vi "potential-field.vi"(10 "Debug":bool=TRUE, 11 "IA State Output in":T1={"our_robots"=[], "enemy_robots"=[], "balls"=[], "geometry"={"line_width"=0, "field_length"=0, "field_width"=0, "boundary_width"=0, "referee_width"=0, "goal_width"=0, "goal_depth"=0, "goal_wall_width"=0, "center_circle_radius"=0, "defense_radius"=0, "defense_stretch"=0, "free_kick_from_defense_dist"=0, "penalty_spot_from_field_line_dist"=0, "penalty_line_from_spot_dist"=0}, "IA Judge"={"stage"="", "command"="", "our_goalie_id"=0.0, "enemy_goalie_id"=0.0, "command enum"=enum."Halt", "Time"=enum."Azul"}, "Received Timestamp"=timestamp(0 s since 1904-01-01), "Events"={"Touch"=FALSE, "Ball out"=FALSE, "id touch"=0.0, "Ball out of \nVision"=FALSE, "Ball inside \nGoalie area"=FALSE, "Robot not responding"=FALSE, "Robots responding status"=[1.0, 1.0, 1.0, 1.0, 1.0, 1.0], "Enemy Ball \nPossession"=FALSE, "Pass State"=FALSE, "id end of pass"=0.0, "Kick"=FALSE, "Id ini Possession"=0.0, "Ball Possesion"=FALSE, "Id Possesion"=0.0}}) -> (3 "IA State Output out":T1={"our_robots"=[], "enemy_robots"=[], "balls"=[], "geometry"={"line_width"=0, "field_length"=0, "field_width"=0, "boundary_width"=0, "referee_width"=0, "goal_width"=0, "goal_depth"=0, "goal_wall_width"=0, "center_circle_radius"=0, "defense_radius"=0, "defense_stretch"=0, "free_kick_from_defense_dist"=0, "penalty_spot_from_field_line_dist"=0, "penalty_line_from_spot_dist"=0}, "IA Judge"={"stage"="", "command"="", "our_goalie_id"=0.0, "enemy_goalie_id"=0.0, "command enum"=enum."Halt", "Time"=enum."Azul"}, "Received Timestamp"=timestamp(0 s since 1904-01-01), "Events"={"Touch"=FALSE, "Ball out"=FALSE, "id touch"=0.0, "Ball out of \nVision"=FALSE, "Ball inside \nGoalie area"=FALSE, "Robot not responding"=FALSE, "Robots responding status"=[1.0, 1.0, 1.0, 1.0, 1.0, 1.0], "Enemy Ball \nPossession"=FALSE, "Pass State"=FALSE, "id end of pass"=0.0, "Kick"=FALSE, "Id ini Possession"=0.0, "Ball Possesion"=FALSE, "Id Possesion"=0.0}})   [LabVIEW 2018]
uses:
  Core/AI Input.ctl
  Core/AI Robot.ctl
  Intel/Functions Enum.ctl
  Intel/AttackerStates.ctl
  Core/AI Ball.ctl
  Core/Field Size.ctl
  Core/AI Judge.ctl
  Intel/Command Enum.ctl
  Util/Events/Events.ctl
  <vilib>/Analysis/_algsub.llb/Vector Norm Type.ctl
  <vilib>/Analysis/_algsub.llb/Real Vector Norm.vi
  <vilib>/Analysis/coordinate.llb/2D Cartesian Coordinate Rotation (Scalar).vi
  <vilib>/Analysis/NI_AALPro.lvlib
panel:
  in  "influence radius":dbl=500.0 format="%#_13g"
  in  "multiplier":dbl(slide)=1.0 scale=0.0..10.0
  in  "dist to nullify pot field":dbl=800.0 format="%#_13g"
  in  "min dist to reduce":dbl=500.0 format="%#_13g"
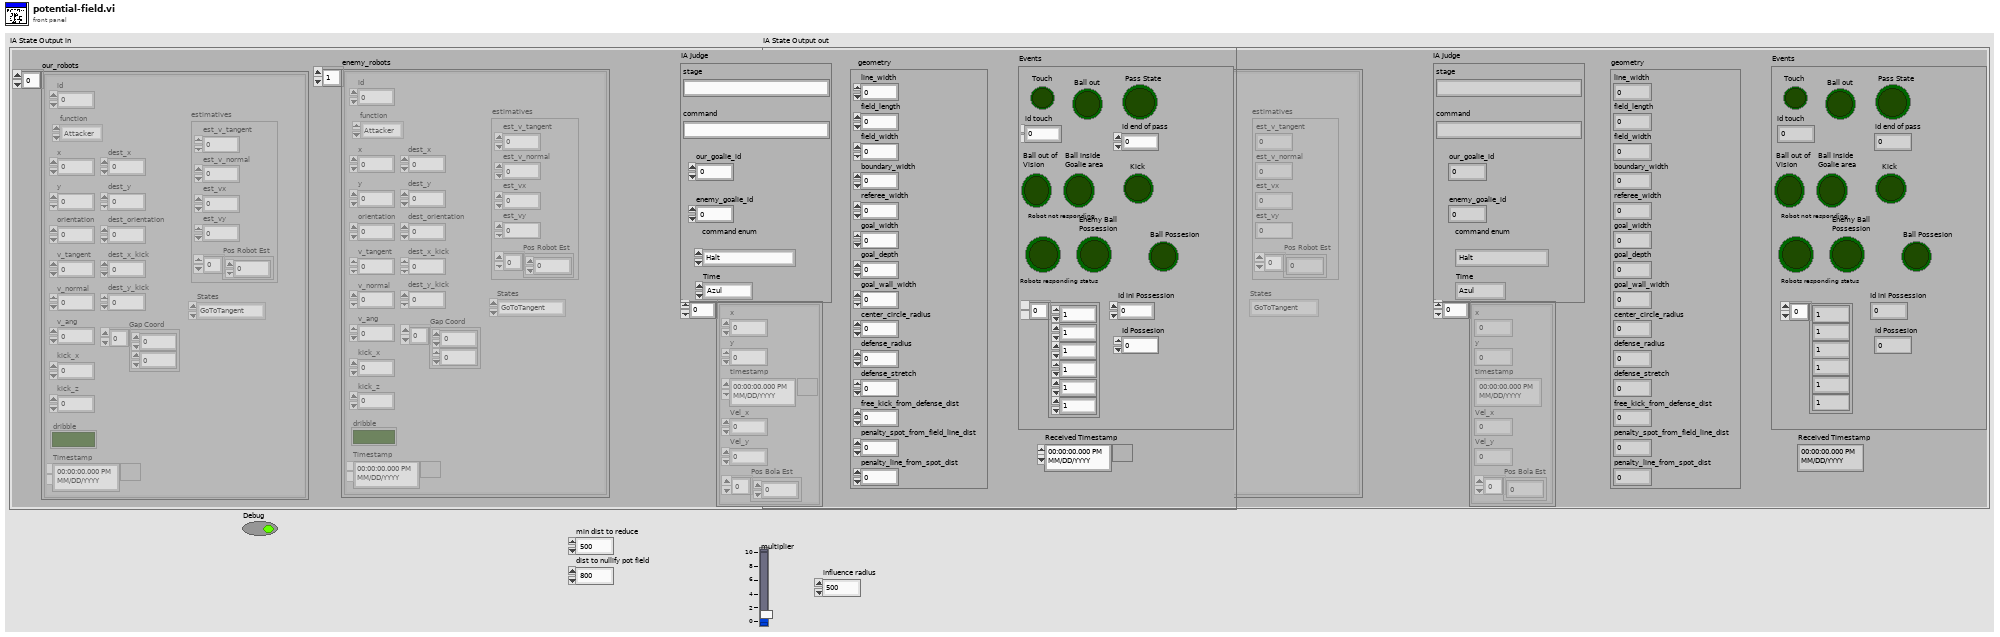
[diagram p1: front panel]
types:
  T1 = typedef "AI Input.ctl" = cluster{"our_robots":T2[], "enemy_robots":T2[], "balls":T5[], "geometry":T6, "IA Judge":T7, "Received Timestamp":timestamp, "Events":T9}
  T2 = typedef "AI Robot.ctl" = cluster{"id":u32, "function":T3, "x":dbl, "y":dbl, "orientation":dbl, "v_tangent":dbl, "v_normal":dbl, "v_ang":dbl, "kick_x":dbl, "kick_z":dbl, "dribble":bool, "Timestamp":timestamp, "dest_x":dbl, "dest_y":dbl, "dest_orientation":dbl, "estimatives":cluster{"est_v_tangent":dbl, "est_v_normal":dbl, "est_vx":dbl, "est_vy":dbl, "Pos Robot Est":dbl[]}, "dest_x_kick":dbl, "dest_y_kick":dbl, "Gap Coord":dbl[], "States":T4}
  T3 = typedef "Functions Enum.ctl" = enum16{"Attacker", "Goalie", "Defender", "Striker", "Goto 0", "Dummy", "Kicker", "ZigZag"}
  T4 = typedef "AttackerStates.ctl" = enum16{"Pass", "GoToTangent", "BallGetting", "GoToKick", ""}
  T5 = typedef "AI Ball.ctl" = cluster{"x":dbl, "y":dbl, "timestamp":timestamp, "Vel_x":dbl, "Vel_y":dbl, "Pos Bola Est":dbl[]}
  T6 = typedef "Field Size.ctl" = cluster{"line_width":u32, "field_length":u32, "field_width":u32, "boundary_width":u32, "referee_width":u32, "goal_width":u32, "goal_depth":u32, "goal_wall_width":u32, "center_circle_radius":u32, "defense_radius":u32, "defense_stretch":u32, "free_kick_from_defense_dist":u32, "penalty_spot_from_field_line_dist":u32, "penalty_line_from_spot_dist":u32}
  T7 = typedef "AI Judge.ctl" = cluster{"stage":string, "command":string, "our_goalie_id":dbl, "enemy_goalie_id":dbl, "command enum":T8, "Time":enum16{"Azul", "Amarelo"}}
  T8 = typedef "Command Enum.ctl" = enum16{"Halt", "Stop", "Force Start", "PKA Normal Start", "Prepare Kickoff Ally", "PKE Normal Start", "Prepare Kickoff Enemy", "Prepare Penalty Ally", "PPA Normal Start", "Prepare Penalty Enemy", "PPE Normal Start", "Direct Free Enemy", "Direct Free Ally", "Indirect Free Enemy", "Indirect Free Ally", "Timeout Enemy", "Timeout Ally", "Goal Enemy", "Goal Ally", "Ball Placement Enemy", "Ball Placement Ally", "Normal Half Time", "Extra Time Break", "Extra Half Time", "None", "Post Game"}
  T9 = typedef "Events.ctl" = cluster{"Touch":bool, "Ball out":bool, "id touch":dbl, "Ball out of \nVision":bool, "Ball inside \nGoalie area":bool, "Robot not responding":bool, "Robots responding status":dbl[], "Enemy Ball \nPossession":bool, "Pass State":bool, "id end of pass":dbl, "Kick":bool, "Id ini Possession":dbl, "Ball Possesion":bool, "Id Possesion":dbl}
  T10 = typedef "NI_AALPro.lvlib/Vector Norm Type.ctl" = u16
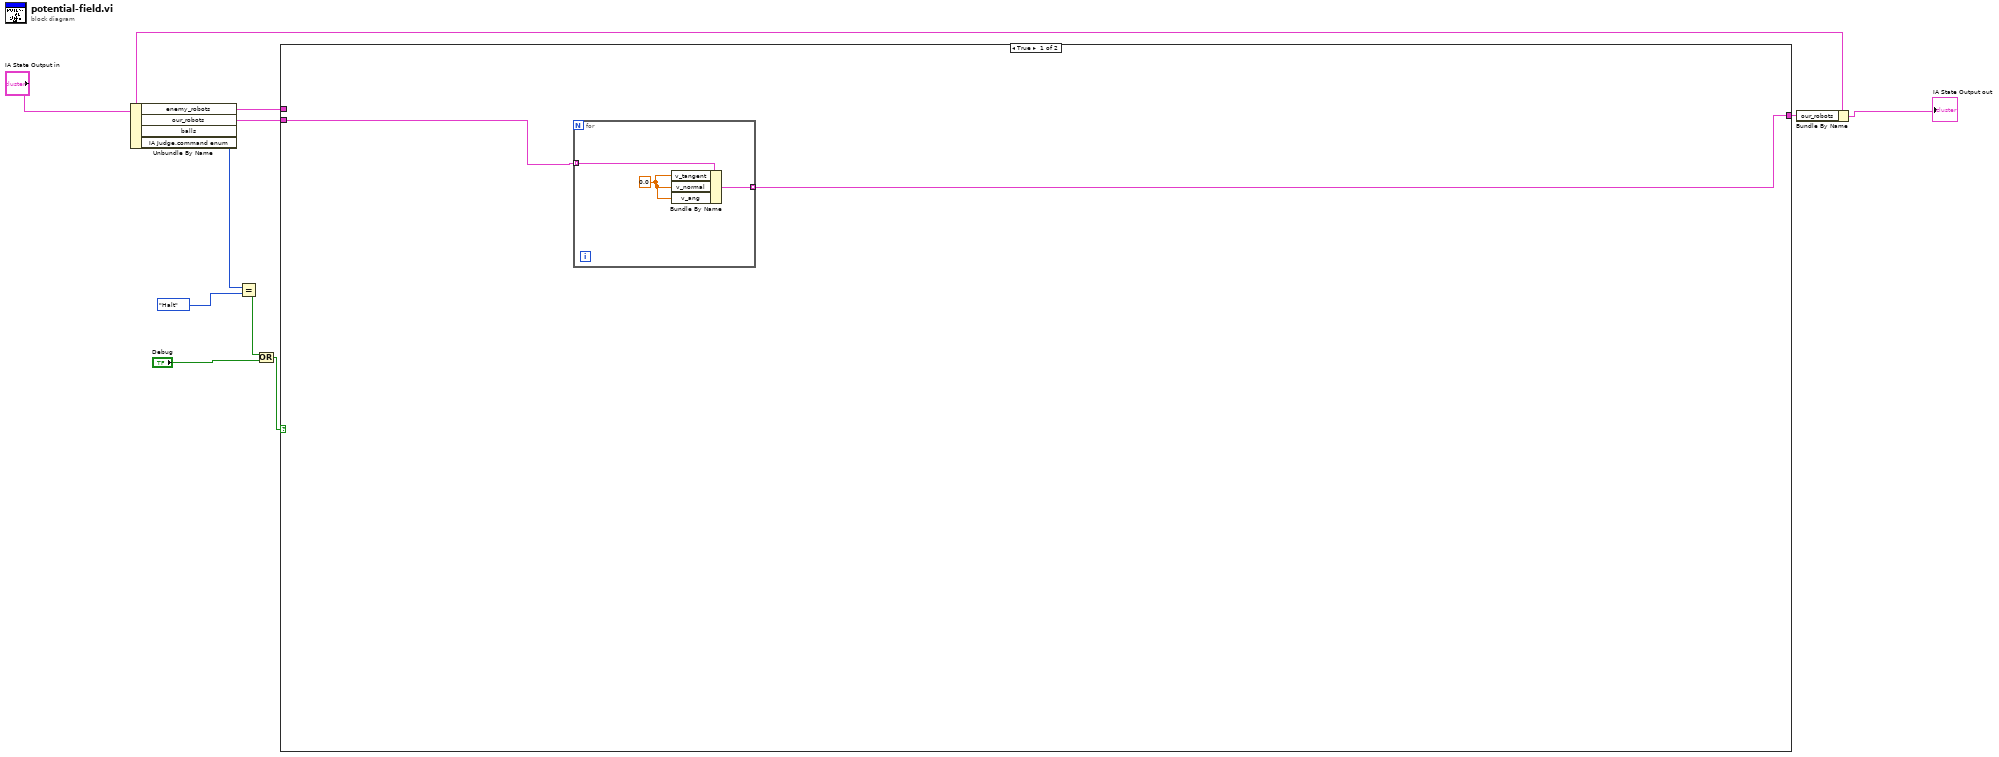
[diagram p0: block diagram]
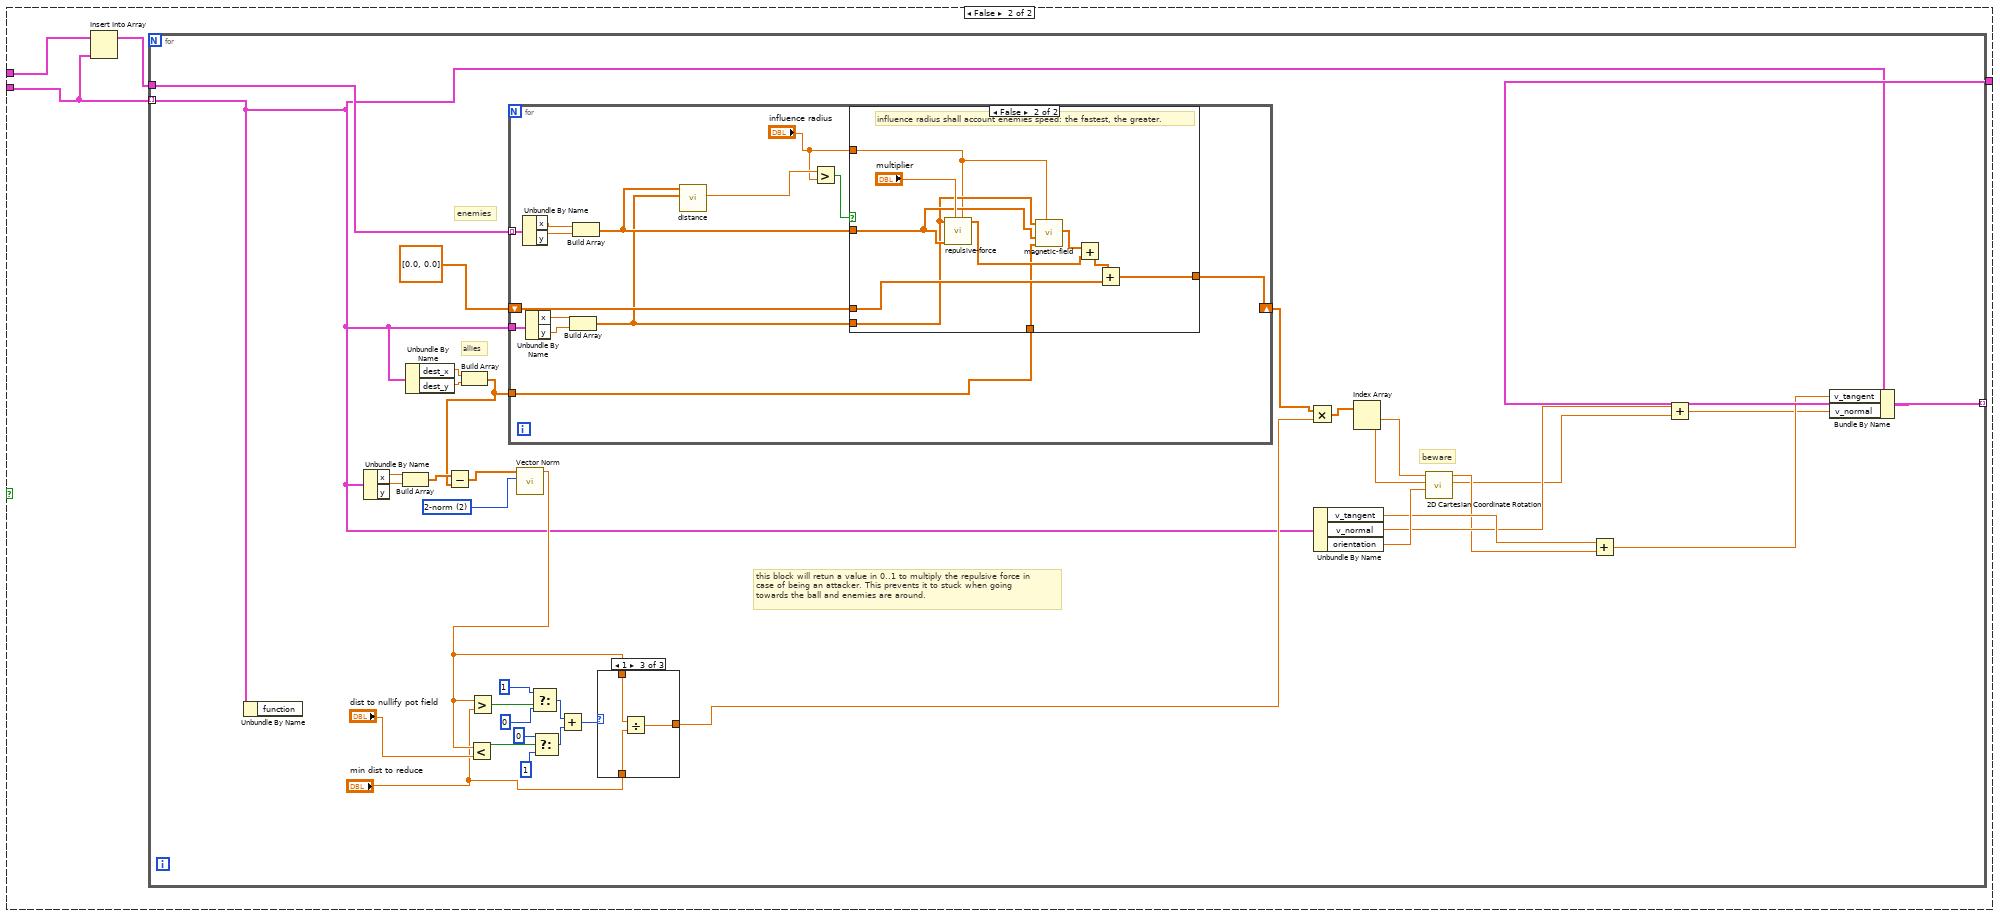
[diagram p2: hidden frame]
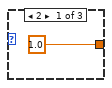
[diagram p3: hidden frame]
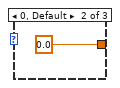
[diagram p4: hidden frame]
diagram:
  n1 = Unbundle By Name("IA State Output in") -> ("enemy_robots"=w10:T2[], "our_robots"=w9:T2[], "IA Judge.command enum"=w5:T8)  [unwired: 1 out]
  n2 = Equal?(x=w5, y=Command_Enum."Halt") -> (x = y?=w2:bool)
  n3 = Or(x=w2, y="Debug") -> (x .or. y?=w1:bool)
  n4 = case shown="True" w1 {
    tunnel: w10 -> [_ w18]
    tunnel: w9 -> [w12 w17]
    tunnel: [w11 w19] -> w8
    frame True {
      n5 = for {
        tunnel: w12 -> [w15] mode=indexing
        tunnel: [w13] -> w11 mode=indexing
        w14 = 0.0
        n6 = Bundle By Name(cluster=w15, "v_tangent"=w14, "v_normal"=w14, "v_ang"=w14) -> (w13:T2)
      }
    }
    frame False {
      n7 = Insert Into Array(array=w18, new element=w17) -> (w16:T2[])  [unwired: 1 in]
      n8 = for {
        tunnel: w16 -> [w55]
        tunnel: w17 -> [w34] mode=indexing
        tunnel: [w45] -> w19 mode=indexing
        w36 = T10 2 items=["1-norm"=1, "2-norm"=2, "Inf-norm"=3, "-Inf-norm"=4, "User Defined"=5] ("norm type")
        # "allies"
        # "enemies"
        # "this block will retun a value in 0..1 to multiply the repulsive force in\ncase of being an attacker. This prevents it to stuck when going \ntowards the ball and enemies are around."
        # "beware"
        n9 = Unbundle By Name(w34) -> ()  [unwired: 1 out]
        n10 = Unbundle By Name(w34) -> ("x"=w40:dbl, "y"=w39:dbl)
        n11 = Build Array(w40, w39) -> (w38:dbl[])
        n12 = Unbundle By Name(w34) -> ("dest_x"=w33:dbl, "dest_y"=w32:dbl)
        n13 = Build Array(w33, w32) -> (w31:dbl[])
        n14 = Subtract(x=w38, y=w31) -> (x-y=w37:dbl[])
        n15 = for {
          tunnel: w55 -> [w74] mode=indexing
          tunnel: w34 -> [w67]
          shift-right: [w68] -> w43
          shift-left: dbl[] [0.0, 0.0] -> [w69]
          tunnel: w31 -> [w64]
          n16 = Unbundle By Name(w74) -> ("x"=w73:dbl, "y"=w72:dbl)
          n17 = Unbundle By Name(w67) -> ("x"=w71:dbl, "y"=w70:dbl)
          n18 = Build Array(w71, w70) -> (w65:dbl[])
          n19 = Build Array(w73, w72) -> (w66:dbl[])
          n20 = call "distance.vi"("target pos"=w65, "obj pos"=w66) -> ("sqrt(x)"=w63:dbl)  [unwired: 9 in]
          n21 = Greater?(x=w63, y="influence radius") -> (0:w61:bool)
          n22 = case shown="False" w61 {
            tunnel: w69 -> [w75 w85]
            tunnel: [w75 w84] -> w68
            tunnel: w66 -> [_ w79]
            tunnel: w65 -> [_ w78]
            tunnel: w64 -> [_ w77]
            tunnel: "influence radius" -> [_ w76]
            frame True {
            }
            frame False {
              # "influence radius shall account enemies speed: the fastest, the greater."
              n23 = call "repulsive-force.vi"("influence radius"=w76, "multiplier"="multiplier", "obstacle pos"=w79, "agent pos"=w78) -> ("force"=w82:dbl[])  [unwired: 6 in, 1 out]
              n24 = call "magnetic-field.vi"("enemy influence radius"=w76, "goal pos"=w77, "enemy pos"=w79, "ally pos"=w78) -> ("magnetic force"=w83:dbl[])  [unwired: 7 in]
              n25 = Add(x=w83, y=w82) -> (x+y=w81:dbl[])
              n26 = Add(x=w81, y=w85) -> (x+y=w84:dbl[])
            }
          }
        }
        n27 = call-poly <vilib>:"Vector Norm.vi"("norm type"=w36, "Input Vector"=w37) -> ("norm"=w35:dbl)  [unwired: 8 in, 1 out]
        n28 = Less?(x=w35, y="dist to nullify pot field") -> (x < y?=w27:bool)
        n29 = Greater?(x=w35, y="min dist to reduce") -> (0:w28:bool)
        n30 = Select(t=1, s=w28, f=0) -> (s? t:f=w29:i32)
        n31 = Select(t=0, s=w27, f=1) -> (s? t:f=w30:i32)
        n32 = Add(x=w29, y=w30) -> (x+y=w21:i32)
        n33 = case shown="1" w21 {
          tunnel: [1.0 0.0 w58] -> w42
          tunnel: w35 -> [_ _ w60]
          tunnel: "min dist to reduce" -> [_ _ w59]
          frame 2 {
          }
          frame 0, Default {
          }
          frame 1 {
            n34 = Divide(x=w60, y=w59) -> (x/y=w58:dbl)
          }
        }
        n35 = Multiply(x=w43, y=w42) -> (x*y=w41:dbl[])
        n36 = Unbundle By Name(w34) -> ("v_tangent"=w51:dbl, "v_normal"=w50:dbl, "orientation"=w52:dbl)
        n37 = Index Array(array=w41) -> (element #1=w54:dbl, element #2=w53:dbl)  [unwired: 2 in]
        n38 = call-poly <vilib>:"2D Cartesian Coordinate Rotation.vi"("theta"=w52, "y"=w53, "x"=w54) -> ("y out"=w48:dbl, "x out"=w49:dbl)  [unwired: 6 in, 1 out]
        n39 = Add(x=w51, y=w49) -> (x+y=w47:dbl)
        n40 = Add(x=w50, y=w48) -> (x+y=w46:dbl)
        n41 = Bundle By Name(cluster=w34, "v_tangent"=w47, "v_normal"=w46) -> (w45:T2)
      }
    }
  }
  n42 = Bundle By Name(cluster="IA State Output in", "our_robots"=w8) -> (→"IA State Output out":T1)
